vi "dotNET Key Management Testing.vi"() -> ()   [LabVIEW 2021]
uses:
  CNG Provider Type.ctl
  CNG Key Info.ctl
  dotNET Crypto Key Management.lvlib
panel:
  in  "Ephemeral key?":bool
  in  "Key Length (2048)":i32=2048
  out "Private Key (Graph)":u8[](graph)
  out "Public Key (Graph)":u8[](graph)
  in  "Machine Key?":bool
  in  "Export Policy (allow export)":i32(ring)=2 items=["None"=0, "AllowExport"=1, "AllowPlaintextExport"=2, "AllowArchiving"=4, "AllowPlaintextArchiving"=8]
  in  "Key Usage (all usages)":i32(ring)=16777215 items=["None"=0, "Decryption"=1, "Signing"=2, "KeyAgreement"=4, "AllUsages"=16777215]
  out "error out":errorcluster
  out "Key Exists?":bool
  out "Public Key":u8[](array[numeric])
  out "Private Key":u8[](array[numeric])
  out "Key Information":T1
  in  "Crypto Provider":T2
  in  "Key Name":string
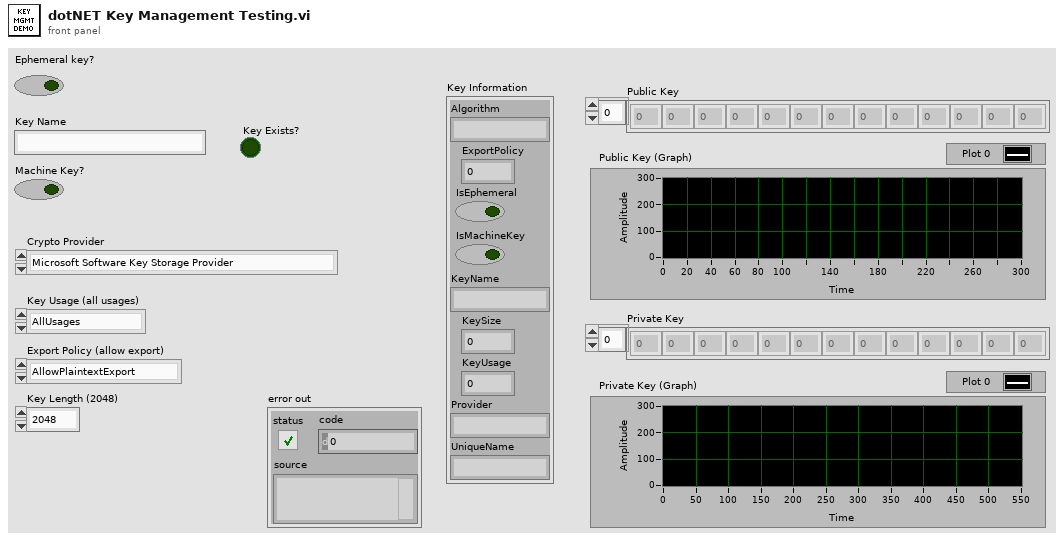
[diagram p1: front panel]
types:
  T1 = typedef "dotNET Crypto Key Management.lvlib/CNG Key Info.ctl" = cluster{"Algorithm":string, "ExportPolicy":i32, "IsEphemeral":bool, "IsMachineKey":bool, "KeyName":string, "KeySize":i32, "KeyUsage":i32, "Provider":string, "UniqueName":string}
  T2 = typedef "dotNET Crypto Key Management.lvlib/CNG Provider Type.ctl" = enum16{"Microsoft Software Key Storage Provider", "Microsoft Platform Crypto Provider"}
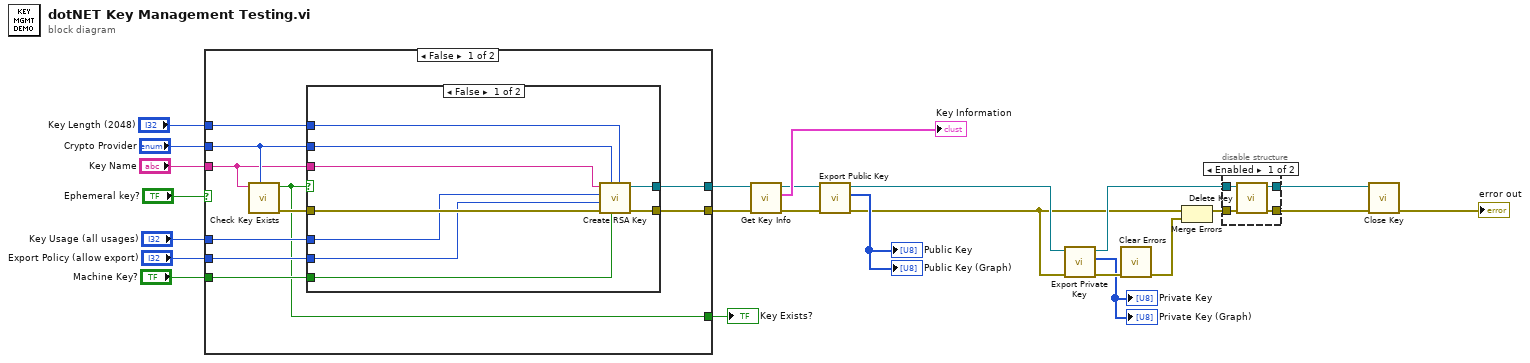
[diagram p0: block diagram]
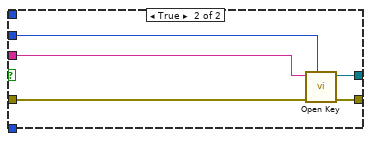
[diagram p2: hidden frame]
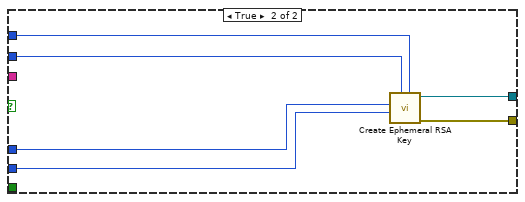
[diagram p3: hidden frame]
diagram:
  n1 = case shown="False" "Ephemeral key?" {
    tunnel: [w33 w54] -> w24
    tunnel: [w32 w53] -> w23
    tunnel: "Crypto Provider" -> [w31 w51]
    tunnel: "Key Name" -> [w30 _]
    tunnel: "Machine Key?" -> [w29 _]
    tunnel: "Export Policy (allow export)" -> [w28 w49]
    tunnel: "Key Usage (all usages)" -> [w27 w50]
    tunnel: "Key Length (2048)" -> [w26 w52]
    tunnel: [w25 _] -> w3
    frame False {
      n2 = call "Check Key Exists.vi"("Crypto Provider"=w31, "Key Name"=w30) -> ("error out"=w34:errorcluster, "Key Exists?"=w25:bool)  [unwired: 8 in]
      n3 = case shown="False" w25 {
        tunnel: w34 -> [w43 w48]
        tunnel: [w42 w47] -> w33
        tunnel: [w41 w46] -> w32
        tunnel: w31 -> [w40 w45]
        tunnel: w30 -> [w39 w44]
        tunnel: w29 -> [w38 _]
        tunnel: w28 -> [w37 _]
        tunnel: w27 -> [w36 _]
        tunnel: w26 -> [w35 _]
        frame False {
          n4 = call "Create RSA Key.vi"("Key Length (2048)"=w35, "Machine Key?"=w38, "Crypto Provider"=w40, "error in (no error)"=w43, "Export Policy (allow export)"=w37, "Key Usage (all usages)"=w36, "Key Name"=w39) -> ("error out"=w42:errorcluster, "CngKey out"=w41:refnum<k24>)  [unwired: 3 in]
        }
        frame True {
          n5 = call "Open Key.vi"("Crypto Provider"=w45, "error in (no error)"=w48, "Key Name"=w44) -> ("error out"=w47:errorcluster, "CngKey out"=w46:refnum<k24>)  [unwired: 7 in]
        }
      }
    }
    frame True {
      n6 = call "Create Ephemeral RSA Key.vi"("Key Length (2048)"=w52, "Crypto Provider"=w51, "Export Policy (allow export)"=w49, "Key Usage (all usages)"=w50) -> ("error out"=w54:errorcluster, "CngKey out"=w53:refnum<k24>)  [unwired: 6 in]
    }
  }
  "Key Exists?" <- w3
  n7 = call "Get Key Info.vi"("error in (no error)"=w24, "CngKey in"=w23) -> ("error out"=w20:errorcluster, "Key Information"=→"Key Information":T1, "CngKey out"=w14:refnum<k24>)  [unwired: 7 in]
  n8 = call "Export Public Key.vi"("error in (no error)"=w20, "CngKey ref in"=w14) -> ("error out"=w11:errorcluster, "Public Key"=→"Public Key" →"Public Key (Graph)":u8[], "CngKey ref out"=w13:refnum<k24>)  [unwired: 7 in]
  n9 = call "Export Private Key.vi"("error in (no error)"=w11, "CngKey ref in"=w13) -> ("error out"=w10:errorcluster, "Private Key"=→"Private Key" →"Private Key (Graph)":u8[], "CngKey ref out"=w17:refnum<k24>)  [unwired: 7 in]
  n10 = call <vilib>:"Clear Errors.vi"("error in (no error)"=w10) -> ("error out"=w8:errorcluster)  [unwired: 5 in, 1 out]
  n11 = Merge Errors(w11, w8) -> (w9:errorcluster)
  n12 = disable-structure shown="Enabled" {
    disable-tunnel: w9 -> [w58 w59]
    disable-tunnel: [w57 w59] -> w18
    disable-tunnel: w17 -> [w56 w60]
    disable-tunnel: [w55 w60] -> w16
    frame Enabled {
      n13 = call "Delete Key.vi"("error in (no error)"=w58, "CngKey in"=w56) -> ("error out"=w57:errorcluster, "CngKey out"=w55:refnum<k24>)  [unwired: 8 in]
    }
    frame Disabled {
    }
  }
  n14 = call "Close Key.vi"("error in (no error)"=w18, "CngKey in"=w16) -> ("error out"=→"error out":errorcluster)  [unwired: 9 in]
